vi "Create From VI Reference.vi"(8 "error in (no error)":errorcluster, 10 "VI":refnum<vi>) -> (0 "error out":errorcluster, 3 "CSM-Helper.lvclass":refnum<class "CSM-Helper.lvclass">)   [LabVIEW 2020, in "CSM-Helper.lvclass"]
uses:
  CSM-Helper.lvclass
  CSM-Helper.lvclass/CSM-Helper.ctl
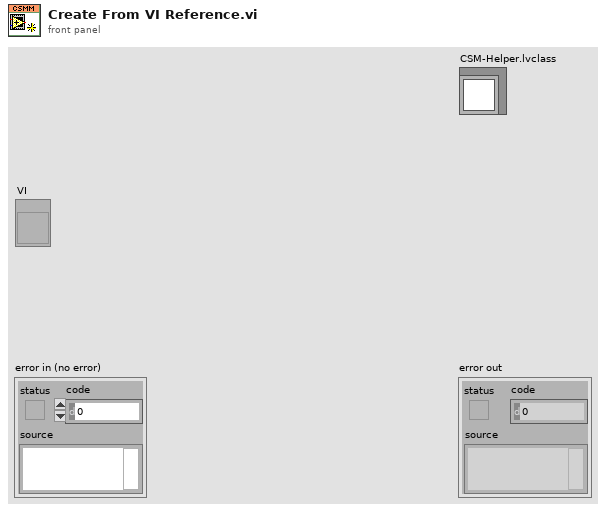
[diagram p1: front panel]
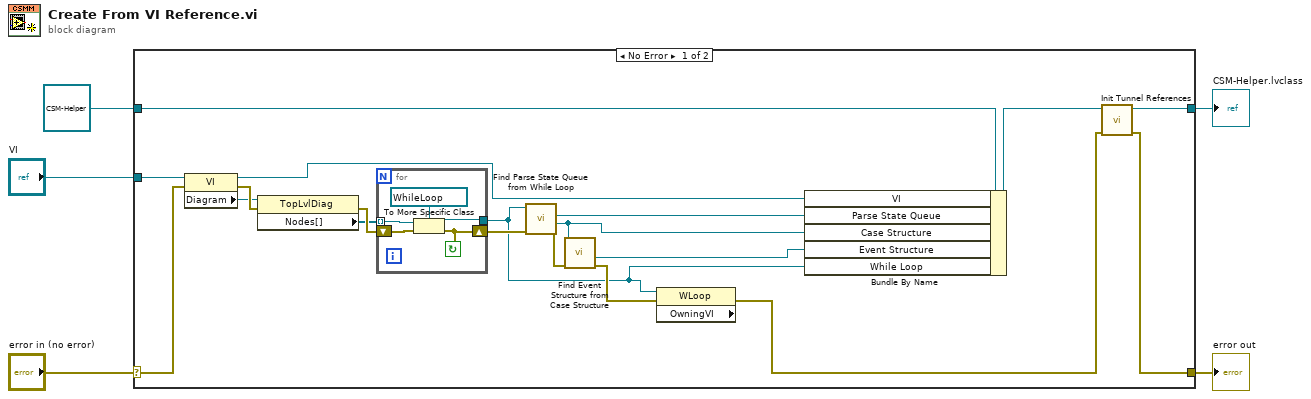
[diagram p0: block diagram]
diagram:
  n1 = case shown="No Error" "error in (no error)" {
    selector: "error in (no error)" -> [w19 w31]
    tunnel: [w9 w31] -> w4
    tunnel: [w11 w30] -> w2
    tunnel: refnum<class "CSM-Helper.lvclass"> refnum ("JKI SM") -> [w18 w30]
    tunnel: "VI" -> [w20 _]
    frame No Error {
      n2 = property class="VI"(reference=w20, error in=w19) -> (reference out=w6:refnum<vi>, error out=w24:errorcluster, "Diagram"=w21:refnum<vi>)
      n3 = property class="TopLvlDiag"(reference=w21, error in=w24) -> (error out=w23:errorcluster, "Nodes[]"=w22:refnum<vi>[])  [unwired: 1 out]
      n4 = for {
        tunnel: w22 -> [w28] mode=indexing
        tunnel: [w26] -> w7
        shift-right: [w25] -> w15
        shift-left: w23 -> [w27]
        stop <- w25 continue-if-true
        n5 = To More Specific Class(target class=refnum<vi> refnum ("WLoop Refnum"), reference=w28, error in=w27) -> (specific class reference=w26:refnum<vi>, error out=w25:errorcluster)
      }
      n6 = call "Find Parse State Queue from While Loop.vi"("error in (no error)"=w15, "WhileLoop in"=w7) -> ("error out"=w16:errorcluster, "CaseStructure"=w14:refnum<vi>, "Parse State Queue"=w17:refnum<vi>)  [unwired: 7 in]
      n7 = call "Find Event Structure from Case Structure.vi"("error in (no error)"=w16, "CaseStructure"=w14) -> ("error out"=w13:errorcluster, "EvntStruct Refnum"=w8:refnum<vi>)  [unwired: 8 in]
      n8 = property class="WLoop" props=["OwningVI"](reference=w7, error in=w13) -> (error out=w10:errorcluster)  [unwired: 2 out]
      n9 = Bundle By Name(cluster=w18, "VI"=w6, "Parse State Queue"=w17, "Case Structure"=w14, "Event Structure"=w8, "While Loop"=w7) -> (w12:refnum<class "CSM-Helper.lvclass">)
      n10 = call "Init Tunnel References.vi"("error in (no error)"=w10, "CSM-Helper in"=w12) -> ("error out"=w9:errorcluster, "CSM-Helper out"=w11:refnum<class "CSM-Helper.lvclass">)  [unwired: 8 in]
    }
    frame Error {
    }
  }
  "error out" <- w4
  "CSM-Helper.lvclass" <- w2
